vi "Create Dictionary from File.vi"(8 "error in":errorcluster, 11 "reference in":refnum<class "Electronic Datasheet.lvclass">) -> (0 "error out":errorcluster, 3 "reference out":refnum<class "Electronic Datasheet.lvclass">)   [LabVIEW 2024, in "Electronic Datasheet.lvlib" / "Electronic Datasheet.lvclass"]
uses:
  Electronic Datasheet/Electronic Datasheet.lvclass
  Electronic Datasheet/Electronic Datasheet.lvclass/Electronic Datasheet.ctl
  <vilib>/Utility/config.llb/NI_LVConfig.lvlib
  Object Dictionary/Dictionary.lvclass
  OD Section/Section.lvclass
  <vilib>/Utility/config.llb/Read Key (String).vi
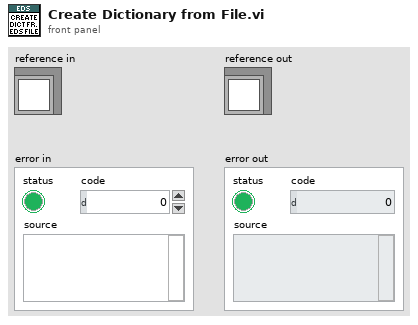
[diagram p1: front panel]
types:
  T1 = typedef "Electronic Datasheet.lvlib/Electronic Datasheet.lvclass/ObjectAttributes.ctl" = cluster{"EDS File Path":path, "Object Dict":refnum<class "Dictionary.lvclass">, "Sorted Object Dict":refnum<class "Sorted Object Dictionary.lvclass">, "Device Info":refnum<class "Device Info.lvclass">, "File Info":refnum<class "File Info.lvclass">}
  T2 = typedef "NI_LVConfig.lvlib/Config Data RefNum.ctl" = refnum<k1>
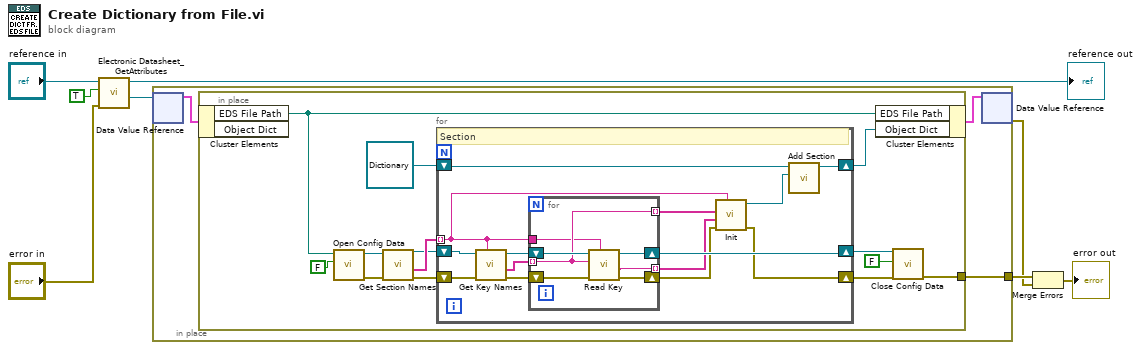
[diagram p0: block diagram]
diagram:
  n1 = call "Electronic Datasheet_GetAttributes.vi"("Error In"="error in", "OnlyGetDvrReference(False)"=TRUE, "reference in"="reference in") -> ("DataRef"=w4:refnum<data-value>, "reference out"=→"reference out":refnum<class "Electronic Datasheet.lvclass">)  [unwired: 5 in, 2 out]
  n2 = in-place {
    in-place-border: [w11] -> w8
    n3 = in-place-dvr #1(w4) -> (w10:T1)  [unwired: 1 out]
    n4 = in-place {
      in-place-border: [w24] -> w11
      n5 = in-place-cluster #2(w10) -> ("EDS File Path"=w13:path)  [unwired: 1 out]
      n6 = call <vilib>:"Open Config Data.vi"("create file if necessary (T)"=FALSE, "configuration file path"=w13) -> ("error out"=w14:errorcluster, "refnum"=w15:T2)  [unwired: 7 in, 1 out]
      n7 = call <vilib>:"Get Section Names.vi"("error in (no error)"=w14, "refnum"=w15) -> ("error out"=w17:errorcluster, "section names"=w22:string[], "refnum out"=w18:T2)  [unwired: 7 in]
      n8 = for {
        tunnel: w22 -> [w30] mode=indexing
        shift-right: [w26] -> w19
        shift-left: w17 -> [w38]
        shift-right: [w34] -> w20
        shift-left: w18 -> [w37]
        shift-right: [w32] -> w12
        shift-left: refnum<class "Dictionary.lvclass"> refnum ("Object Dictionary") -> [w31]
        # "Section"
        n9 = call <vilib>:"Get Key Names.vi"("section"=w30, "error in (no error)"=w38, "refnum"=w37) -> ("error out"=w36:errorcluster, "key names"=w33:string[], "refnum out"=w35:T2)  [unwired: 5 in, 1 out]
        n10 = for {
          shift-right: [w41] -> w27
          shift-left: w36 -> [w45]
          tunnel: w33 -> [w40] mode=indexing
          shift-right: [w43] -> w34
          shift-left: w35 -> [w44]
          tunnel: [w42] -> w28 mode=indexing
          tunnel: [w40] -> w29 mode=indexing
          tunnel: w30 -> [w39]
          n11 = call-poly <vilib>:"Read Key.vi"("section"=w39, "error in (no error)"=w45, "key"=w40, "refnum"=w44) -> ("error out"=w41:errorcluster, "value"=w42:string, "refnum out"=w43:T2)  [unwired: 4 in, 1 out]
        }
        n12 = call "Init.vi"("Name"=w30, "error in"=w27, "Values"=w28, "Keynames"=w29) -> ("error out"=w26:errorcluster, "Section out"=w25:refnum<class "Section.lvclass">)  [unwired: 6 in]
        n13 = call "Add Section.vi"("Section"=w25, "Dictionary in"=w31) -> ("Dictionary out"=w32:refnum<class "Dictionary.lvclass">)  [unwired: 9 in]
      }
      n14 = in-place-cluster #2("EDS File Path"=w13, "Object Dict"=w12) -> (w9:T1)
      n15 = call <vilib>:"Close Config Data.vi"("error in (no error)"=w19, "write file if changed (T)"=FALSE, "refnum"=w20) -> ("error out"=w24:errorcluster)  [unwired: 7 in, 1 out]
    }
    n16 = in-place-dvr #1(w9) -> (w1:errorcluster)  [unwired: 1 out]
  }
  n17 = Merge Errors(w8, w1) -> (→"error out":errorcluster)
